vi "Read Timeout.vi"(8 "error in (no error)":errorcluster, 11 "Lamp in":refnum<class "Lamp.lvclass">) -> (0 "error out":errorcluster, 2 "Timeout":dbl, 3 "Lamp out":refnum<class "Lamp.lvclass">)   [LabVIEW 2016, in "Lamp.lvclass"]
uses:
  Lamp.lvclass
  Lamp.lvclass/Lamp.ctl
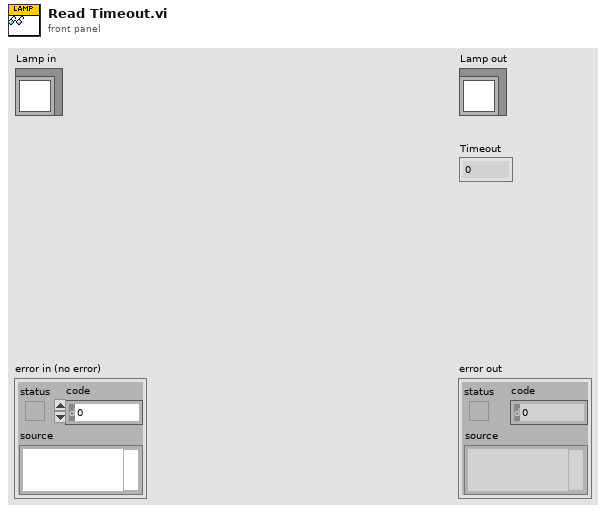
[diagram p1: front panel]
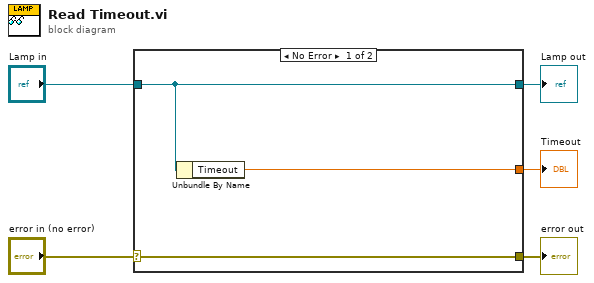
[diagram p0: block diagram]
diagram:
  n1 = case shown="No Error" "error in (no error)" {
    selector: "error in (no error)" -> [w8 w9]
    tunnel: [w8 w9] -> w4
    tunnel: [w7 w10] -> w2
    tunnel: "Lamp in" -> [w7 w10]
    tunnel: [w6 _] -> w1
    frame No Error {
      n2 = Unbundle By Name(w7) -> ("Timeout"=w6:dbl)
    }
    frame Error {
    }
  }
  "error out" <- w4
  "Lamp out" <- w2
  "Timeout" <- w1
